vi "Difference Quotient (single).vi"(6 "Interval Units (points)":enum16{"Points", "Data"}(ring), 8 "error in (no error)":errorcluster, 9 "Type":enum16{"y/x vs x", "x/y vs y"}(ring), 10 "Window [h] (2)":dbl=2.0, 11 "XY-data":cluster{"X-array":dbl[], "Y-array":dbl[]}) -> (0 "error out":errorcluster, 2 "Difference Quotient":cluster{"X-array":dbl[], "Y-array":dbl[]} {"Y-array" format="%.2p"; "X-array" format="%.2p"}, 3 "XY-data out":cluster{"X-array":dbl[], "Y-array":dbl[]})   [LabVIEW 2019, in "xy_utilities.lvlib"]
doc: "Calculate the difference quotient (y[i-h/2]-y[i+h/s])/(x[i-h/2]-x[i+h/2]).\n\nWire data to the data input to determine the polymorphic instance to use or manually select the instance."
uses:
  xy_utilities.lvlib
  Swap X and Y (single).vi
  Reverse (single).vi
  Divide float (single).vi
  Add XY (single).vi
  Private/X Array Range to Index.vi
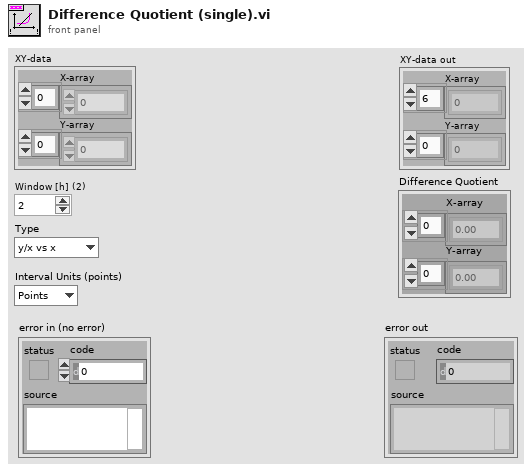
[diagram p1: front panel]
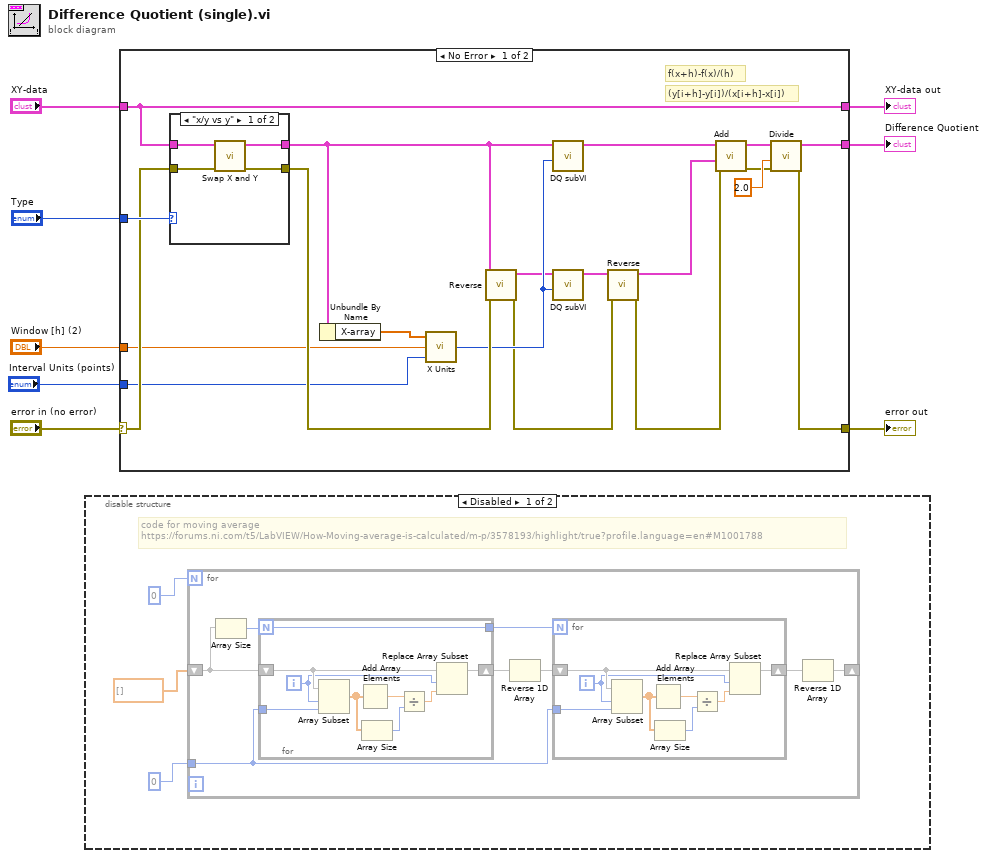
[diagram p0: block diagram]
diagram:
  n1 = disable-structure shown="Disabled" {
    frame Disabled {
      # "code for moving average\nhttps://forums.ni.com/t5/LabVIEW/How-Moving-average-is-calculated/m-p/3578193/highlight/true?profile.language=en#M1001788"
      n2 = for {
        N: 0 ("iterations") -> [_]
        tunnel: 0 ("Window") -> [w15]
        shift-right: [w14] -> _
        shift-left: dbl[] [] ("Data In") -> [w19]
        n3 = Array Size(array=w19) -> (size(s)=w13:i32)
        n4 = for {
          N: w13 -> [w28]
          shift-right: [w32] -> w18
          shift-left: w19 -> [w35]
          tunnel: w15 -> [w31]
          tunnel: [w28] -> w12
          i -> [w34]
          n5 = Array Subset(array=w35, index=w34, length=w31) -> (w30:dbl[])
          n6 = Add Array Elements(numeric array=w30) -> (sum=w36:dbl)
          n7 = Array Size(array=w30) -> (size(s)=w29:i32)
          n8 = Divide(x=w36, y=w29) -> (x/y=w33:dbl)
          n9 = Replace Array Subset(array=w35, new element=w33, index=w34) -> (w32:dbl[])
        }
        n10 = Reverse 1D Array(array=w18) -> (reversed array=w17:dbl[])
        n11 = for {
          N: w12 -> [_]
          shift-right: [w23] -> w16
          shift-left: w17 -> [w26]
          tunnel: w15 -> [w22]
          i -> [w25]
          n12 = Array Subset(array=w26, index=w25, length=w22) -> (w21:dbl[])
          n13 = Add Array Elements(numeric array=w21) -> (sum=w27:dbl)
          n14 = Array Size(array=w21) -> (size(s)=w20:i32)
          n15 = Divide(x=w27, y=w20) -> (x/y=w24:dbl)
          n16 = Replace Array Subset(array=w26, new element=w24, index=w25) -> (w23:dbl[])
        }
        n17 = Reverse 1D Array(array=w16) -> (reversed array=w14:dbl[])
      }
    }
    frame Enabled {
    }
  }
  n18 = case shown="No Error" "error in (no error)" {
    selector: "error in (no error)" -> [w55 w64]
    tunnel: [w50 w64] -> w7
    tunnel: "XY-data" -> [w54 w63]
    tunnel: [w52 _] -> w5
    tunnel: "Type" -> [w56 _]
    tunnel: [w54 w63] -> w3
    tunnel: "Window [h] (2)" -> [w48 _]
    tunnel: "Interval Units (points)" -> [w47 _]
    frame No Error {
      # "(y[i+h]-y[i])/(x[i+h]-x[i])"
      # "f(x+h)-f(x)/(h)"
      n19 = case shown="\"x/y vs y\"" w56 {
        tunnel: w54 -> [w60 w62]
        tunnel: [w59 w62] -> w53
        tunnel: [w58 w61] -> w51
        tunnel: w55 -> [w57 w61]
        frame "x/y vs y" {
          n20 = call-poly "Swap X and Y.vi"("error in (no error)"=w57, "XY-data"=w60) -> ("error out"=w58:errorcluster, "XY-data out"=w59:cluster{"X-array":dbl[], "Y-array":dbl[]})  [unwired: 8 in]
        }
        frame "y/x vs x" {
        }
      }
      n21 = Unbundle By Name(w53) -> ("X-array"=w49:dbl[])
      n22 = call "X Units.vi"("Interval Units (points)"=w47, "Interval (h)"=w48, "X-array"=w49) -> ("h (points)"=w46:i32)
      n23 = call-poly "Reverse.vi"("error in (no error)"=w51, "XY-data"=w53) -> ("error out"=w41:errorcluster, "Reversed XY-data out"=w45:cluster{"X-array":dbl[], "Y-array":dbl[]})  [unwired: 8 in]
      n24 = call "DQ subVI.vi"("window (h)"=w46, "XY-data"=w53) -> ("XY-data"=w38:cluster{"X-array":dbl[], "Y-array":dbl[]})  [unwired: 9 in]
      n25 = call "DQ subVI.vi"("window (h)"=w46, "XY-data"=w45) -> ("XY-data"=w44:cluster{"X-array":dbl[], "Y-array":dbl[]})  [unwired: 9 in]
      n26 = call-poly "Reverse.vi"("error in (no error)"=w41, "XY-data"=w44) -> ("error out"=w39:errorcluster, "Reversed XY-data out"=w37:cluster{"X-array":dbl[], "Y-array":dbl[]})  [unwired: 8 in]
      n27 = call-poly "Add.vi"("error in (no error)"=w39, "y"=w37, "XY-data"=w38) -> ("error out"=w40:errorcluster, "XY-data out"=w43:cluster{"X-array":dbl[], "Y-array":dbl[]})  [unwired: 7 in]
      n28 = call-poly "Divide.vi"("error in (no error)"=w40, "y (1)"=2.0, "XY-data"=w43) -> ("error out"=w50:errorcluster, "XY-data out"=w52:cluster{"X-array":dbl[], "Y-array":dbl[]})  [unwired: 7 in]
    }
    frame Error {
    }
  }
  "error out" <- w7
  "Difference Quotient" <- w5
  "XY-data out" <- w3
